vi "Current VI's Path (VI or exe).vi"() -> (6 "Full Path to VI or executable":path, 10 "VI or executable installation directory":path)   [LabVIEW 2016]
doc: "Current VI's Path (VI or exe).vi\n\n<B>Description:</B>\n\nThe Current VI's Path (VI or exe) VI is a drop-in replacement for the native Current VI's Path function. Just replace the native Current VI's Path function in your application with the Current VI's Path (VI or exe) VI and you'll never have to deal with the frustration caused by bad paths again -- whether you run your code in the development environment or as an executable!\n\nThe Current VI's Path (VI or exe) VI gets the path to the VI that called it and searches that path for \".exe\". If \".exe\" is found in the path, then the Current VI's Path (VI or exe) VI strips the path twice to obtain the executable's installation directory. If \".exe\" is not found, then the Current VI's Path (VI or exe) VI strips the path once to obtain the VI's installation directory.\n\nIn either case, the Current VI's Path (VI or exe) VI returns the VI or executable installation directory and the Full Path to the VI or executable. You can use this information in your application to easily access sub folders of the VI's or executable's installation directory by using the Build Path function to append the sub directory's name to the VI's or executable's installation path returned by the Current VI's Path (VI or exe) VI.\n\n<B>Usage:</B>\n\nUse the Current VI's Path (VI or exe) VI wherever you would use the native Current VI's Path function.\n\n<B>NOTES:</B>\n\nNone.\n\n<B>Inputs:</B>\n\nNone.\n\n<B>Outputs:</B>\n\nFull Path to VI or executable - The full path to the VI or executable.\n\nVI or executable installation directory - The path to the installation directory of the VI or executable.\n\n<B>Developed by:</B>\n\nMark Ridgley\nmark.ridgley@logicpd.com"
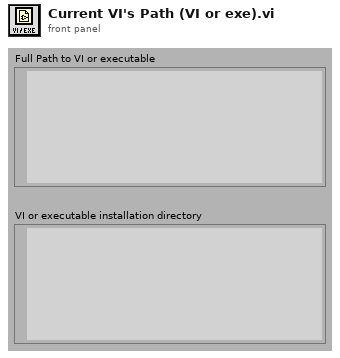
[diagram p1: front panel]
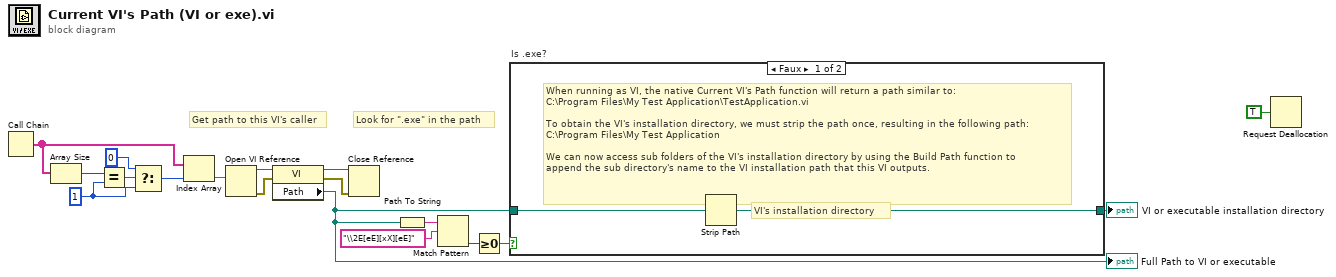
[diagram p0: block diagram]
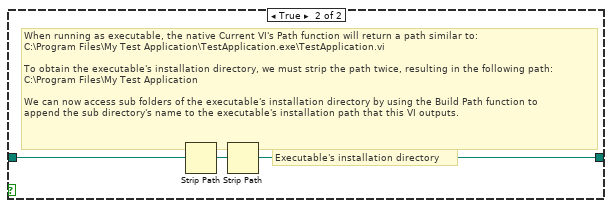
[diagram p2: hidden frame]
diagram:
  w9 = 1 ("index")
  # "Get path to this VI's caller"
  # "Look for \".exe\" in the path"
  n1 = Call Chain() -> (call chain=w13:string[])
  n2 = Array Size(array=w13) -> (size(s)=w10:i32)
  n3 = Equal?(x=w10, y=w9) -> (x = y?=w12:bool)
  n4 = Select(t=0, s=w12, f=w9) -> (s? t:f=w11:i32)
  n5 = Index Array(array=w13, index=w11) -> (element=w5:string)
  n6 = Open VI Reference(vi path=w5) -> (vi reference=w6:refnum<vi>, error out=w7:errorcluster)  [unwired: 5 in]
  n7 = property class="VI"(reference=w6, error in=w7) -> (reference out=w2:refnum<vi>, error out=w3:errorcluster, "Path"=w4:path)
  "Full Path to VI or executable" <- w4
  n8 = Close Reference(reference=w2, error in (no error)=w3) -> ()  [unwired: 1 out]
  n9 = Path To String(path=w4) -> (string=w15:string)
  n10 = Match Pattern(string=w15, regular expression="\\2E[eE][xX][eE]") -> (offset past match=w17:i32)  [unwired: 1 in, 3 out]
  n11 = Greater Or Equal To 0?(x=w17) -> (x >= 0?=w16:bool)
  n12 = case "Is .exe?" shown="Faux" w16 {
    tunnel: w4 -> [w20 w23]
    tunnel: [w19 w21] -> w18
    frame False {
      # "VI's installation directory"
      # "When running as VI, the native Current VI's Path function will return a path similar to:\nC:\\Program Files\\My Test Application\\TestApplication.vi\n\nTo obtain the VI's installation directory, we must strip the path once, resulting in the following path:\nC:\\Program Files\\My Test Application\n\nWe can now access sub folders of the VI's installation directory by using the Build Path function to\nappend the sub directory's name to the VI installation path that this VI outputs."
      n13 = Strip Path(path=w20) -> (stripped path=w19:path)  [unwired: 1 out]
    }
    frame True {
      # "Executable's installation directory"
      # "When running as executable, the native Current VI's Path function will return a path similar to:\nC:\\Program Files\\My Test Application\\TestApplication.exe\\TestApplication.vi\n\nTo obtain the executable's installation directory, we must strip the path twice, resulting in the following path:\nC:\\Program Files\\My Test Application\n\nWe can now access sub folders of the executable's installation directory by using the Build Path function to\nappend the sub directory's name to the executable's installation path that this VI outputs."
      n14 = Strip Path(path=w23) -> (stripped path=w22:path)  [unwired: 1 out]
      n15 = Strip Path(path=w22) -> (stripped path=w21:path)  [unwired: 1 out]
    }
  }
  "VI or executable installation directory" <- w18
  n16 = Request Deallocation(TRUE ("flag")) -> ()
